vi "Global terminating.vi"() -> ()   [LabVIEW 2012]
panel:
  in  "terminating?":bool
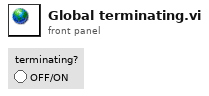
[diagram p1: front panel]
diagram:
